vi "Main.vi"() -> ()   [LabVIEW 2024]
doc: "Event-driven Queue State Machine (EDQSM) template in LabVIEW, designed to manage states and data via a queue. It includes three subVIs to create, enqueue, and dequeue states with attached data (using Variant for flexibility). The functional example features a simple interface with buttons that trigger events. The template is easily transformable into a traditional Queue State Machine (QSM) by removing the Wait state."
uses:
  controls/Data.ctl
  support/queue state & data (Array).vi
  <vilib>/Utility/error.llb/Error Cluster From Error Code.vi
  support/queue state & data (Single).vi
  <vilib>/ErrorRing/Error Ring.xnode
  support/queue state & data.lvlib
panel:
  in  "Run Test 2":bool
  in  "Run Test 1":bool
  in  "Stop Button":bool
  # "State Machine (State & Data)"
  # "Improving string-based State Machine"
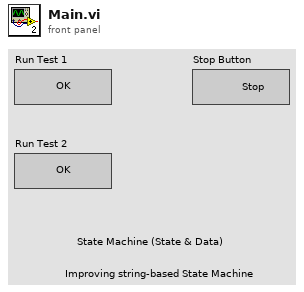
[diagram p1: front panel]
types:
  T1 = typedef "Data.ctl" = cluster{"Boolean":bool, "String":string, "Numeric":dbl, "Run Test1 Ref":refnum<vi>, "Run Test2 Ref":refnum<vi>, "Stop Butt Ref":refnum<vi>}
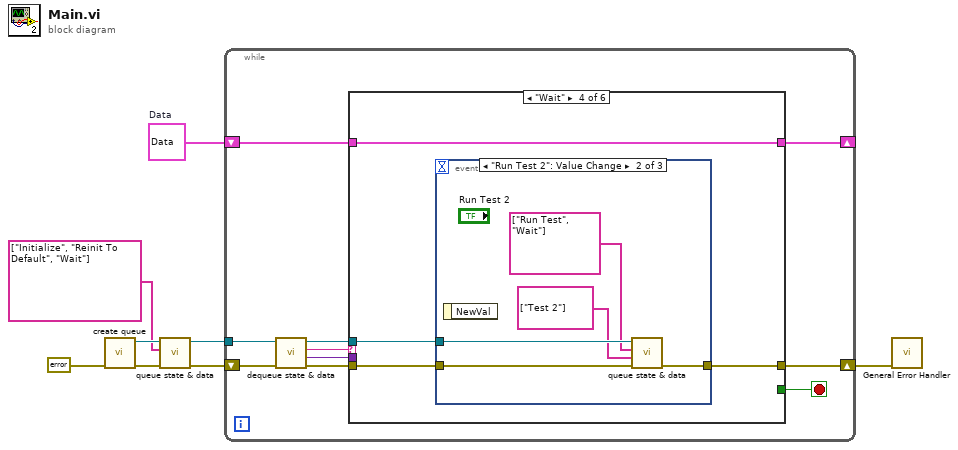
[diagram p0: block diagram]
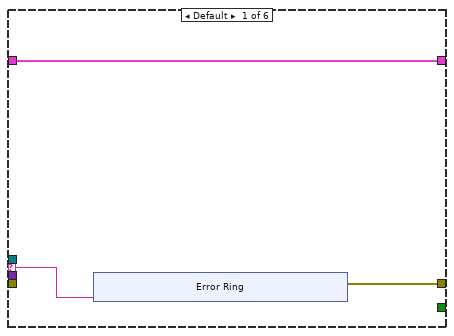
[diagram p2: hidden frame]
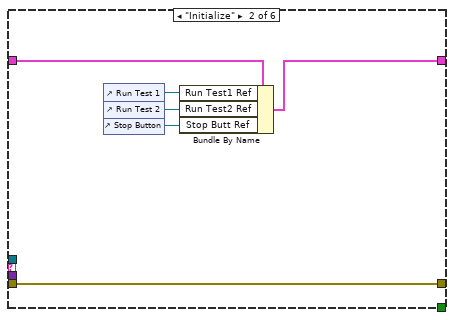
[diagram p3: hidden frame]
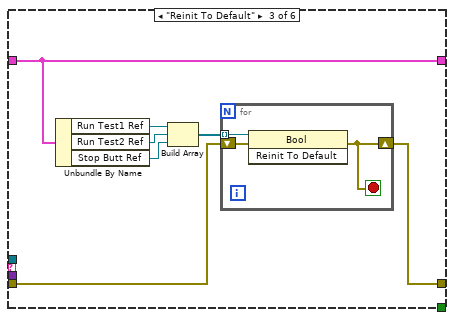
[diagram p4: hidden frame]
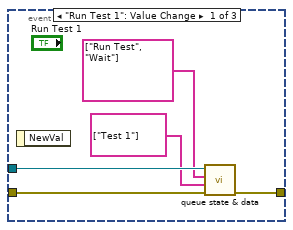
[diagram p5: hidden frame]
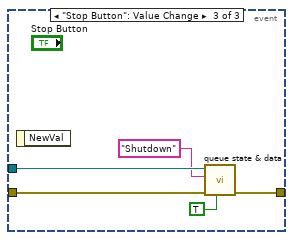
[diagram p6: hidden frame]
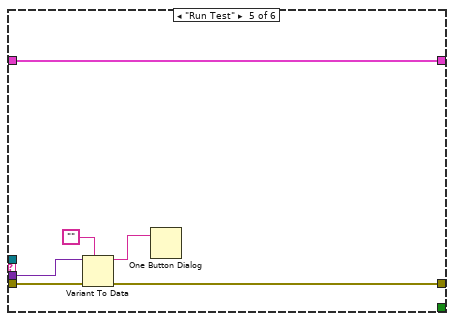
[diagram p7: hidden frame]
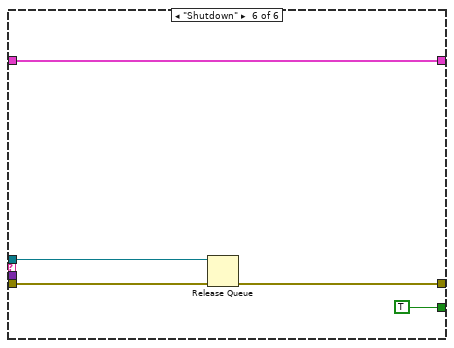
[diagram p8: hidden frame]
diagram:
  w3 = T1 {"Boolean"=FALSE, "String"="", "Numeric"=0.0, "Run Test1 Ref"=refnum, "Run Test2 Ref"=refnum, "Stop Butt Ref"=refnum}  # Data
  n1 = call "create queue.vi"("error in (no error)"=errorcluster {"status"=FALSE, "code"=0, "source"=""} ("error constant")) -> ("error out"=w5:errorcluster, "queue out"=w7:refnum<queue>)  [unwired: 9 in]
  n2 = call-poly "queue state & data.vi"("error in (no error)"=w5, "State Array"=string[] ["Initialize", "Reinit To Default", "Wait"], "queue in"=w7) -> ("error out"=w6:errorcluster, "queue out"=w4:refnum<queue>)  [unwired: 7 in]
  n3 = while {
    shift-right: [w18] -> w8
    shift-left: w6 -> [w13]
    tunnel: w4 -> [w11]
    shift-right: [w9] -> _
    shift-left: w3 -> [w10]
    stop <- w17 stop-if-true
    n4 = call "dequeue state & data.vi"("error in (no error)"=w13, "queue in"=w11) -> ("error out"=w16:errorcluster, "State Data"=w14:variant, "State"=w15:string, "queue out"=w12:refnum<queue>)  [unwired: 6 in]
    n5 = case shown="\"Wait\"" w15 {
      selector: w15 -> [w20 _ _ _ _ _]
      tunnel: w16 -> [_ w29 w36 w48 w69 w73]
      tunnel: [w21 w29 w35 w47 w68 w71] -> w18
      tunnel: [_ _ _ _ _ TRUE] -> w17
      tunnel: w12 -> [_ _ _ w46 _ w72]
      tunnel: w14 -> [_ _ _ _ w67 _]
      tunnel: w10 -> [w19 w34 w41 w45 w64 w70]
      tunnel: [w19 w33 w41 w45 w64 w70] -> w9
      frame Default {
        n6 = xnode ("Error Ring")("parameter 0"=w20) -> ("error out"=w21:errorcluster)
      }
      frame "Initialize" {
        n7 = control-ref of="Run Test 1"() -> (w32:refnum<vi>)
        n8 = control-ref of="Run Test 2"() -> (w31:refnum<vi>)
        n9 = control-ref of="Stop Button"() -> (w30:refnum<vi>)
        n10 = Bundle By Name(cluster=w34, "Run Test1 Ref"=w32, "Run Test2 Ref"=w31, "Stop Butt Ref"=w30) -> (w33:T1)
      }
      frame "Reinit To Default" {
        n11 = Unbundle By Name(w41) -> ("Run Test1 Ref"=w40:refnum<vi>, "Run Test2 Ref"=w39:refnum<vi>, "Stop Butt Ref"=w38:refnum<vi>)
        n12 = Build Array(w40, w39, w38) -> (w37:refnum<vi>[])
        n13 = for {
          tunnel: w37 -> [w44] mode=indexing
          shift-right: [w42] -> w35
          shift-left: w36 -> [w43]
          stop <- w42 stop-if-true
          n14 = invoke on="Invoke Node" class="Bool" method="Reinit To Default"(reference=w44, error in=w43) -> (error out=w42:errorcluster)  [unwired: 1 in, 2 out]
        }
      }
      frame "Wait" {
        n15 = event shown="[1] \"Run Test 2\": Value Change" {
          selector: _ -> [_ _ _]
          dyn-events: _ -> [_ _ _]
          timeout: _ -> [_ _ _]
          tunnel: w48 -> [w53 w58 w62]
          tunnel: [w52 w57 w63] -> w47
          tunnel: w46 -> [w51 w56 w61]
          event "Run Test 1": Value Change {
            n16 = event-data() -> ()  [unwired: 1 in, 1 out]
            n17 = call-poly "queue state & data.vi"("error in (no error)"=w53, "State Data Array"=string[] ["Test 1"], "State Array"=string[] ["Run Test", "Wait"], "queue in"=w51) -> ("error out"=w52:errorcluster)  [unwired: 6 in, 1 out]
          }
          event "Run Test 2": Value Change {
            n18 = event-data() -> ()  [unwired: 1 in, 1 out]
            n19 = call-poly "queue state & data.vi"("error in (no error)"=w58, "State Data Array"=string[] ["Test 2"], "State Array"=string[] ["Run Test", "Wait"], "queue in"=w56) -> ("error out"=w57:errorcluster)  [unwired: 6 in, 1 out]
          }
          event "Stop Button": Value Change {
            n20 = event-data() -> ()  [unwired: 1 in, 1 out]
            n21 = call-poly "queue state & data.vi"("Priority State? (F)"=TRUE ("Priority? (F)"), "error in (no error)"=w62, "State"="Shutdown", "queue in"=w61) -> ("error out"=w63:errorcluster)  [unwired: 6 in, 1 out]
          }
        }
      }
      frame "Run Test" {
        n22 = Variant To Data(error in=w69, type="" ("Empty String Constant"), Variant=w67) -> (data=w65:string, error out=w68:errorcluster)
        n23 = One Button Dialog(message=w65) -> ()  [unwired: 1 in, 1 out]
      }
      frame "Shutdown" {
        n24 = Release Queue(queue=w72, error in (no error)=w73) -> (error out=w71:errorcluster)  [unwired: 1 in, 2 out]
      }
    }
  }
  n25 = call <vilib>:"General Error Handler.vi"("error in (no error)"=w8) -> ()  [unwired: 10 in, 5 out]
